vi "3.STM Basic Server.vi"() -> ()   [LabVIEW 2014]
doc: "This example demonstrates how to implement a STM server which sends messages to the client.\n\nThe server needs to be started before the client."
uses:
  vi.lib/Q-WaveSystems/QwaveSys Raspberry Pi for LabVIEW Home-Education/STM/_SubVIs/stm_MetaDataElement.ctl
  vi.lib/Q-WaveSystems/QwaveSys Raspberry Pi for LabVIEW Home-Education/STM/TCP/STM Write Meta Data (TCP Ref).vi
  vi.lib/Q-WaveSystems/QwaveSys Raspberry Pi for LabVIEW Home-Education/STM/TCP/STM Write Message (TCP).vi
  vi.lib/Q-WaveSystems/QwaveSys Raspberry Pi for LabVIEW Home-Education/STM/TCP/STM Get Connection Reference (TCP).vi
  vi.lib/Q-WaveSystems/QwaveSys Raspberry Pi for LabVIEW Home-Education/QwaveSys Raspberry Pi Library.lvlib
panel:
  out "error out":errorcluster
  in  "stop":bool
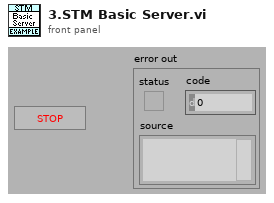
[diagram p1: front panel]
types:
  T1 = typedef "QwaveSys Raspberry Pi Library.lvlib/stm_MetaDataElement.ctl" = string
  T2 = typedef "QwaveSys Raspberry Pi Library.lvlib/stm_TCP Connection Info.ctl" = cluster{"connection ID":refnum<k5>, "Meta data":T1[]}
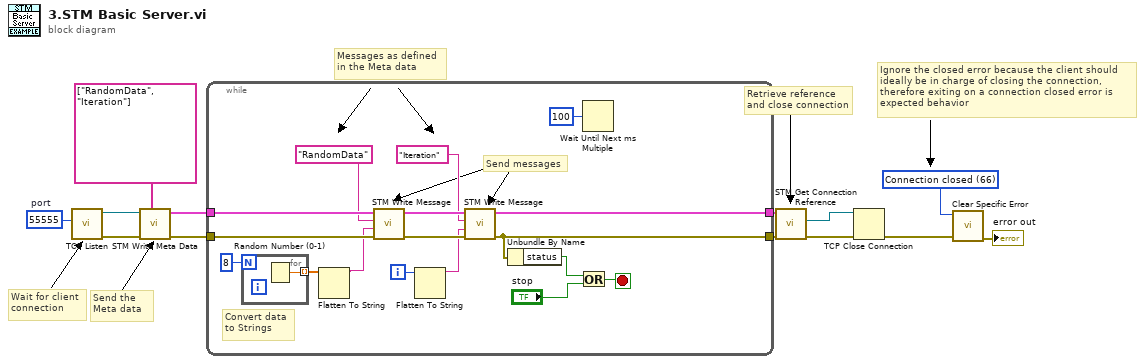
[diagram p0: block diagram]
diagram:
  w8 = 66 items=["No Error", "Argument Error", "Memory Full", "Out of Zone", "End of File", "File Already Open", "Generic File IO Error", "File Not Found", "File Permission Error", "Disk Full", "Duplicate Path", "Too Many Files Open", "Not Enabled", "Resource File Not Found", "Cannot Add Resource", "Resource Not Found", "Image Not Found", "Image Memory Error", "Pen Does Not Exist", "Config Bad Type", "Config Token Not Found", "Config Parse Error", "Config Memory Error", "Bad External Code Format", "Bad External Code Offset", "External Code Not Present", "Null Window", "Destroy Window Mixup", "Null Menu", "Print Aborted", "Bad Print Record", "Print Driver Error", "Windows Error During Print", "Memory Error During Print", "Print Dialog Error", "Generic Print Error", "Invalid Device Refnum", "Device Not Found", "Device Parameter Error", "Device Unit Error", "Can't Open Device", "Device Call Aborted", "Generic Error", "Cancelled By User", "Object ID Too Low", "Object ID Too High", "Object Not In Heap", "Unknown Heap", "Bad DefProc ID", "DefProc Not In Table", "Message Out Of Range", "Null Method", "Unknown Message", "Manager Call Not Supported", "Bad address", "Connection In progress", "Connection timed out", "Connection is already in progress", "Network attribute not supported", "Network error", "Address in use", "System out of memory", "Connection aborted", "Connection refused", "Connection is not connected", "Connection is already connected", "Connection closed", "Initialize error (interapplication manager)", "Bad occurrence", "Wait on unbound occurrence handler", "Occurrence queue overflow", "Bad path", "Semaphore not signaled", "Unrecognized type (interapplication manager)"] ("1st Error to Convert")
  w13 = u16 55555  # port
  # "Ignore the closed error because the client should ideally be in charge of closing the connection, therefore exiting on a connection closed error is expected behavior"
  # "Retrieve reference and close connection"
  # "Meta data"
  # "Messages as defined\nin the Meta data"
  # "Wait for client\nconnection"
  # "Send the\nMeta data"
  n1 = call <vilib>:"TCP Listen.vi"("port"=w13) -> ("error out"=w11:errorcluster, "connection ID"=w12:refnum<k5>)  [unwired: 3 in, 6 out]
  n2 = call-poly "STM Write Meta Data.vi"("Meta data"=T1[] ["RandomData", "Iteration"], "error in"=w11, "connection ID"=w12) -> ("error out"=w9:errorcluster, "Connection Info Out"=w10:T2)  [unwired: 1 in, 6 out]
  n3 = while {
    tunnel: w10 -> [w30]
    tunnel: w9 -> [w29]
    tunnel: [w28] -> w5
    tunnel: [w21] -> w3
    i -> [w17]
    stop <- w22 stop-if-true
    # "Send messages"
    # "Convert data\nto Strings"
    n4 = for {
      N: 8 -> [_]
      tunnel: [w31] -> w18 mode=indexing
      n5 = Random Number (0-1)() -> (number: 0 to 1=w31:dbl)
    }
    n6 = Flatten To String(anything=w18) -> (data string=w15:string)  [unwired: 1 in, 4 out]
    n7 = call-poly "STM Write Message.vi"("error in (no error)"=w29, "Data"=w15, "Name"="RandomData", "Connection Info"=w30) -> ("error out"=w27:errorcluster, "Connection Info Out"=w26:T2)  [unwired: 1 in, 5 out]
    n8 = Flatten To String(anything=w17) -> (data string=w16:string)  [unwired: 1 in, 4 out]
    n9 = call-poly "STM Write Message.vi"("error in (no error)"=w27, "Data"=w16, "Name"="Iteration", "Connection Info"=w26) -> ("error out"=w21:errorcluster, "Connection Info Out"=w28:T2)  [unwired: 1 in, 5 out]
    n10 = Unbundle By Name(w21) -> ("status"=w20:bool)
    n11 = Or(x=w20, y="stop") -> (x .or. y?=w22:bool)
    n12 = Wait Until Next ms Multiple(millisecond multiple=u32 100) -> ()  [unwired: 1 out]
  }
  n13 = call-poly "STM Get Connection Reference.vi"("error in"=w3, "Connection Info"=w5) -> ("error out"=w2:errorcluster, "connection ID out"=w4:refnum<k5>)  [unwired: 8 out]
  n14 = TCP Close Connection(connection ID=w4, error in (no error)=w2) -> (error out=w7:errorcluster)  [unwired: 2 out]
  n15 = call "Clear Specific Error.vi"("error in (no error)"=w7, "code"=w8) -> ("error out"=→"error out":errorcluster)  [unwired: 9 out]
